vi "LP-sctl-3.vi"(6 "Ready For Output":bool, 7 "reset":bool, 8 "Input Valid":bool, 9 "param":T1={"base freq (Hz)"=[20123.0, 20123.0, 20123.0], "P gain"=[1234.0, 1234.0, 1234.0], "I gain"=[1.0, 1.0, 1.0], "LP1 coeffs"=[-1025014616, 2098093632, 165702, -1053286467, 2126356551, 167935, -1025014616, 2098093632, 165702, -1053286467, 2126356551, 167935, -1025014616, 2098093632, 165702, -1053286467, 2126356551, 167935], "scope on"=FALSE, "scope channel"=0, "scope signal"=0, "notch coeff"=[-1025014616, 2098093632, 165702, -1053286467, 2126356551, 167935, -1025014616, 2098093632, 165702]}, 10 "Y in":fxp<+/-,16,2>, 11 "X in":fxp<+/-,16,2>) -> (0 "Output Valid":bool, 2 "Y out":fxp<+/-,16,1> format="%.16g", 3 "X out":fxp<+/-,16,1> format="%.16g", 4 "Ready For Input":bool=TRUE)   [LabVIEW 2018, in "SCTL.lvlib"]
doc: "This VI is used in four wire handshake."
uses:
  SCTL.lvlib
  param-sctl-pll.ctl
panel:
  # "Inputs"
  # "Outputs"
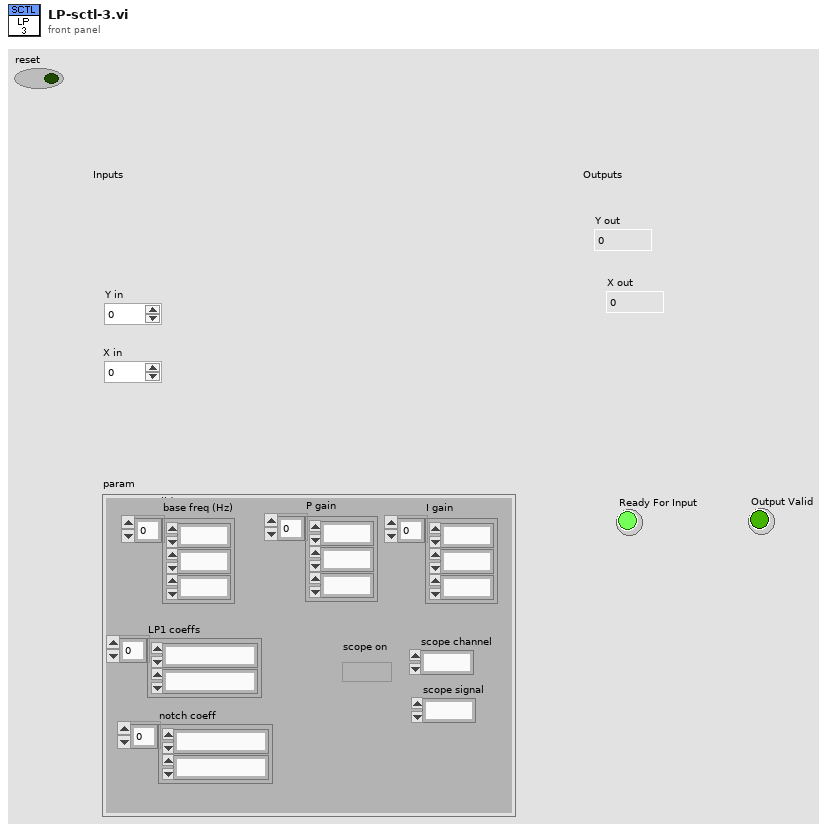
[diagram p1: front panel]
types:
  T1 = typedef "SCTL.lvlib/param-sctl-pll.ctl" = cluster{"base freq (Hz)":fxp<+,17,17>[], "P gain":fxp<+,14,14>[], "I gain":fxp<+,20,6>[], "LP1 coeffs":i32[], "scope on":bool, "scope channel":u8, "scope signal":u8, "notch coeff":i32[]}
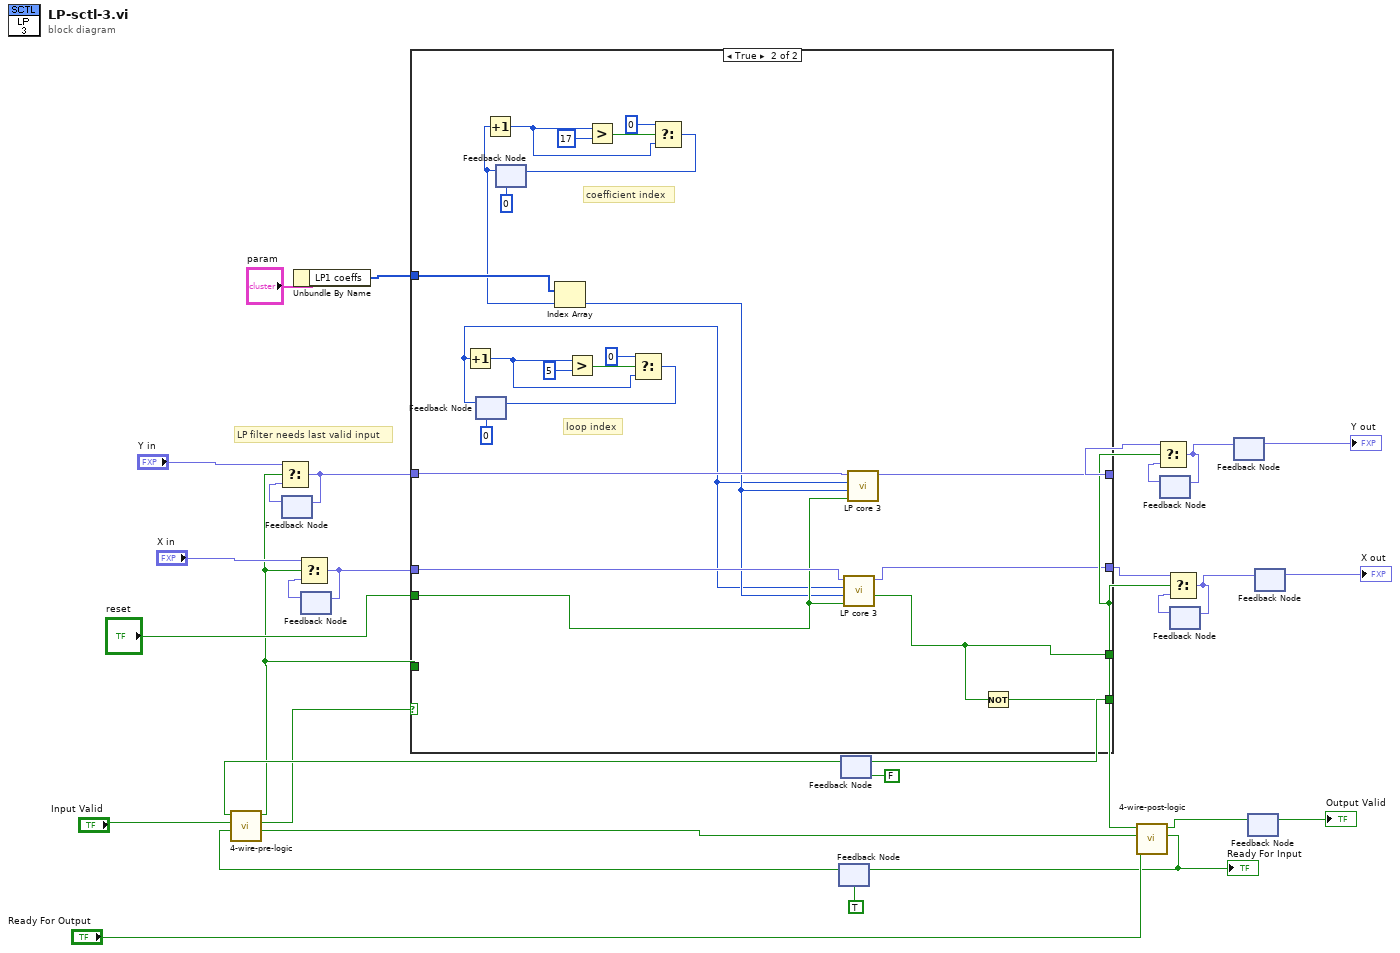
[diagram p0: block diagram]
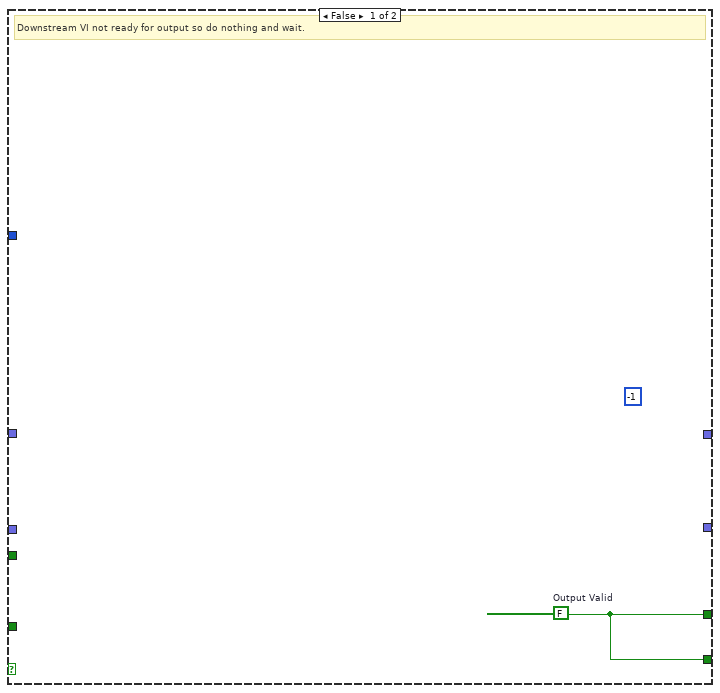
[diagram p2: hidden frame]
diagram:
  # "LP filter needs last valid input"
  n1 = feedback #1() -> (w11:fxp<+/-,16,2>)  [unwired: 1 in]
  n2 = Unbundle By Name("param") -> ("LP1 coeffs"=w1:i32[])
  n3 = feedback #2() -> (w20:fxp<+/-,16,2>)  [unwired: 1 in]
  n4 = feedback #3(TRUE ("x .and. y?")) -> (w29:bool)
  n5 = feedback #4(FALSE ("x .and. y?")) -> (w27:bool)
  n6 = call "4-wire-pre-logic.vi"("ready for input in"=w29, "Input Valid in"="Input Valid", "needs more iter in"=w27) -> ("register state out"=w30:bool, "excecute"=w26:bool, "buffer input!"=w8:bool)  [unwired: 6 in]
  n7 = Select(t="Y in", s=w8, f=w11) -> (s? t:f=w9:fxp<+/-,16,2>)
  n8 = feedback-in #1(w9) -> ()
  n9 = Select(t="X in", s=w8, f=w20) -> (s? t:f=w18:fxp<+/-,16,2>)
  n10 = feedback-in #2(w18) -> ()
  n11 = case shown="True" w26 {
    tunnel: [w32 w53] -> w12
    tunnel: w8 -> [_ _]
    tunnel: [w32 w52] -> w25
    tunnel: w18 -> [_ w55]
    tunnel: [_ w54] -> w16
    tunnel: "reset" -> [_ w51]
    tunnel: [_ w50] -> w13
    tunnel: w9 -> [_ w49]
    tunnel: w1 -> [_ w40]
    frame False {
      (unwired) i16 -1 ("index")
      w32 = FALSE  # Output Valid
      # "Downstream VI not ready for output so do nothing and wait."
    }
    frame True {
      # "coefficient index"
      # "loop index"
      n12 = feedback #5(i16 0) -> (w42:i16)
      n13 = Increment(x=w42) -> (x+1=w45:i16)
      n14 = feedback #6(i16 0) -> (w33:i16)
      n15 = Increment(x=w33) -> (x+1=w36:i16)
      n16 = Index Array(array=w40, index=w33) -> (element=w43:i32)
      n17 = Greater?(x=w45, y=i16 5) -> (0:w41:bool)
      n18 = Greater?(x=w36, y=i16 17) -> (0:w34:bool)
      n19 = Select(t=i16 0, s=w41, f=w45) -> (s? t:f=w44:i16)
      n20 = feedback-in #5(w44) -> ()
      n21 = Select(t=i16 0, s=w34, f=w36) -> (s? t:f=w35:i16)
      n22 = feedback-in #6(w35) -> ()
      n23 = call "LP core 3.vi"("reset"=w51, "coeff"=w43, "index"=w42, "data in"=w55) -> ("output valid!"=w53:bool, "data out"=w54:fxp<+/-,16,1>)  [unwired: 6 in]
      n24 = call "LP core 3.vi"("reset"=w51, "coeff"=w43, "index"=w42, "data in"=w49) -> ("data out"=w50:fxp<+/-,16,1>)  [unwired: 6 in, 1 out]
      n25 = Not(x=w53) -> (.not. x?=w52:bool)
    }
  }
  n26 = feedback-in #4(w25) -> ()
  n27 = call "4-wire-post-logic.vi"("Ready For Output in"="Ready For Output", "register state in"=w30, "output valid in"=w12) -> ("ready for input out"=w22:bool, "output valid out"=w21:bool)  [unwired: 7 in]
  "Ready For Input" <- w22
  n28 = feedback-in #3(w22) -> ()
  n29 = feedback #7() -> (w6:fxp<+/-,16,1>)  [unwired: 1 in]
  n30 = Select(t=w13, s=w12, f=w6) -> (s? t:f=w14:fxp<+/-,16,1>)
  n31 = feedback-in #7(w14) -> ()
  n32 = feedback #8() -> (w7:fxp<+/-,16,1>)  [unwired: 1 in]
  n33 = Select(t=w16, s=w12, f=w7) -> (s? t:f=w17:fxp<+/-,16,1>)
  n34 = feedback-in #8(w17) -> ()
  n35 = feedback-in #9(w14) -> ()
  n36 = feedback #9() -> (→"Y out":fxp<+/-,16,1>)  [unwired: 1 in]
  n37 = feedback-in #10(w21) -> ()
  n38 = feedback #10() -> (→"Output Valid":bool)  [unwired: 1 in]
  n39 = feedback-in #11(w17) -> ()
  n40 = feedback #11() -> (→"X out":fxp<+/-,16,1>)  [unwired: 1 in]
